vi "test_OneSessTwoPinOneInstrOneSiteReservation_VISAGetConnectionsNPinsMConnections_ReturnsThreeConnections.vi"(8 "error in":errorcluster) -> (0 "error out":errorcluster, 2 "result":string, 3 "pass":bool)   [LabVIEW 2020, in "MeasurementServerTests.lvlib"]
uses:
  MeasurementServerTests.lvlib
  Runtime/Measurement Plugin Session Management V1/Session Reservation/Connection.ctl
  Runtime/Measurement Plugin Session Management V1/Session Reservation/Session Reservation.lvclass
  03fc85e1-696b-4ece-a78b-f41470766ac0.vi
  a536e905-e99b-4ce6-9f7b-add65bd26abc.vi
  f2d0f46c-20cf-4e81-b3a3-5c4fc317eda1.vi
  Runtime/Sessions/VISA Sessions/VISA Sessions.lvlib
  Runtime/Sessions/VISA Sessions/Get Connections - NPin MConn.vi
  Runtime/Sessions/VISA Sessions/Connection with Session.ctl
  bf3d92c7-31a5-48e7-a722-05fd9bdeea10.vi
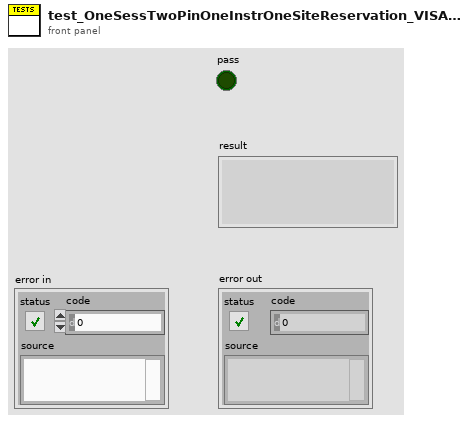
[diagram p1: front panel]
types:
  T1 = typedef "Measurement Plugin Session Management V1.lvlib/Session Reservation.lvclass/Connection.ctl" = cluster{"pin or relay name":string, "site":i32, "instrument type id":string, "channel":string}
  T2 = typedef "VISA Sessions.lvlib/Connection with Session.ctl" = cluster{"connection":T1, "session":refnum<visa-resource-name>}
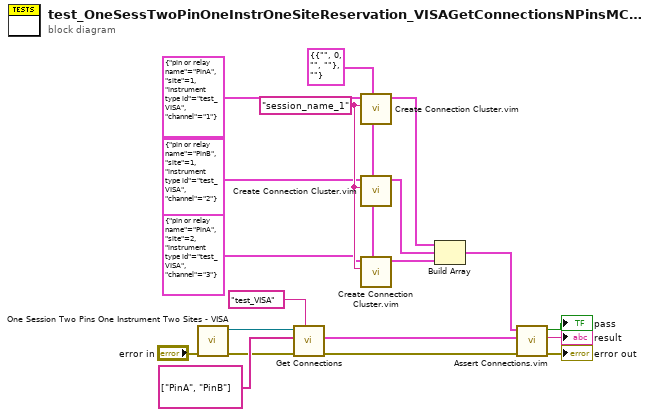
[diagram p0: block diagram]
diagram:
  w9 = T2 {"connection"={"pin or relay name"="", "site"=0, "instrument type id"="", "channel"=""}, "session"=""} ("niDCPower connection")
  w10 = "session_name_1" ("session in")
  n1 = call "One Session Two Pins One Instrument Two Sites - VISA.vi"("error in"="error in") -> ("error out"=w5:errorcluster, "session reservation out"=w4:refnum<class "Session Reservation.lvclass">)  [unwired: 9 in]
  n2 = call-poly "Get Connections.vi"("instrument type id"="test_VISA", "error in"=w5, "pin or relay names"=string[] ["PinA", "PinB"], "session reservation in"=w4) -> ("error out"=w2:errorcluster, "connections"=w19:T2[])  [unwired: 5 in, 1 out]
  n3 = call "Create Connection Cluster.vim"("connection type"=w9, "session in"=w10, "hardware independent connection in"=T1 {"pin or relay name"="PinA", "site"=1, "instrument type id"="test_VISA", "channel"="1"} ("connection")) -> ("connection out"=w14:T2)  [unwired: 8 in]
  n4 = call "Create Connection Cluster.vim"("connection type"=w9, "session in"=w10, "hardware independent connection in"=T1 {"pin or relay name"="PinB", "site"=1, "instrument type id"="test_VISA", "channel"="2"} ("connection")) -> ("connection out"=w13:T2)  [unwired: 8 in]
  n5 = call "Create Connection Cluster.vim"("connection type"=w9, "session in"=w10, "hardware independent connection in"=T1 {"pin or relay name"="PinA", "site"=2, "instrument type id"="test_VISA", "channel"="3"} ("connection")) -> ("connection out"=w8:T2)  [unwired: 8 in]
  n6 = Build Array(w14, w13, w8) -> (w12:T2[])
  n7 = call "Assert Connections.vim"("error in"=w2, "actual connections"=w19, "expected connections"=w12) -> ("error out"=→"error out":errorcluster, "result"=→"result":string, "pass"=→"pass":bool)  [unwired: 6 in]
